vi "abcBuilder.vi"() -> (3 "Array":cluster{string, string}[](array[cluster]))   [LabVIEW 2017]
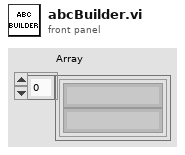
[diagram p1: front panel]
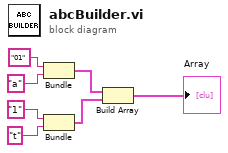
[diagram p0: block diagram]
diagram:
  n1 = Bundle("01", "a") -> (w4:cluster{string, string})  [unwired: 1 in]
  n2 = Bundle("1", "t") -> (w5:cluster{string, string})  [unwired: 1 in]
  n3 = Build Array(w4, w5) -> (→"Array":cluster{string, string}[])
